vi "Endpoint.vi"(6 "abort (F)":bool, 9 "element in":bool) -> (0 "missed":i32, 1 "element out":bool, 3 "channel out":T1, 4 "aborted?":bool)   [LabVIEW 2020, in "Tag-bool.lvlib"]
uses:
  <extravilib>/ChannelInstances/Tag-bool.lvlib
  <extravilib>/ChannelInstances/Tag-bool/))Channel.ctl
  <extravilib>/ChannelInstances/Tag-bool/ChannelOp.ctl
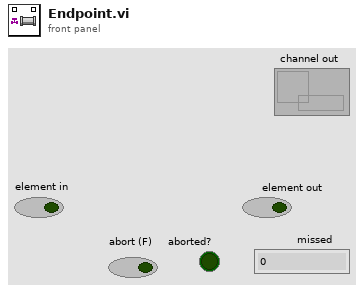
[diagram p1: front panel]
types:
  T1 = typedef "Tag-bool.lvlib/))Channel.ctl" = refnum<queue>
  T2 = typedef "Tag-bool.lvlib/ChannelOp.ctl" = enum16{"init", "write", "read", "probe"}
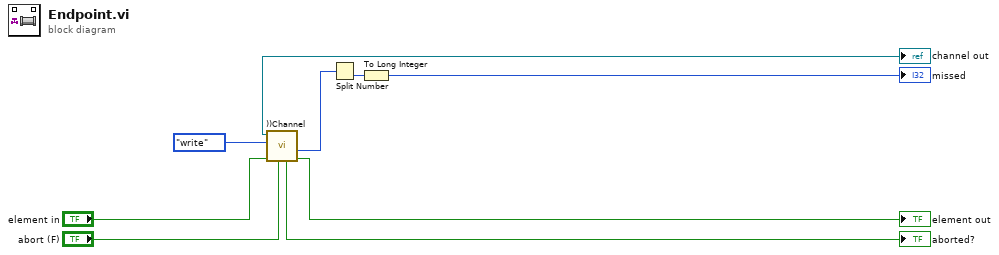
[diagram p0: block diagram]
diagram:
  n1 = call <extravilib>:"))Channel.vi"("abort (F)"="abort (F)", "element in"="element in", "channelOp"=ChannelOp."write", "channel in"="channel out") -> ("element out"=→"element out":bool, "sequence"=w3:u64, "aborted?"=→"aborted?":bool)  [unwired: 2 in, 3 out]
  n2 = Split Number(x=w3) -> (lo(x)=w1:u32)  [unwired: 1 out]
  n3 = To Long Integer(number=w1) -> (32bit integer=→"missed":i32)
